vi "Alternating LEDs.vi"() -> ()   [LabVIEW 2014]
panel:
  in  "stop":bool
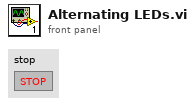
[diagram p1: front panel]
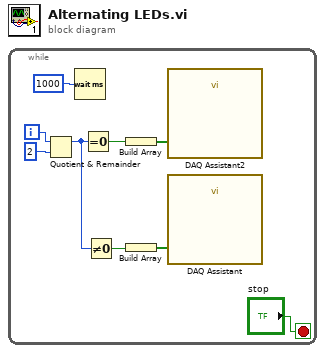
[diagram p0: block diagram]
diagram:
  n1 = while {
    i -> [w9]
    stop <- "stop" stop-if-true
    n2 = Quotient & Remainder(x=w9, y=2) -> (x-y*floor(x/y)=w3:i32)  [unwired: 1 out]
    n3 = Wait (ms)(milliseconds to wait=1000) -> ()  [unwired: 1 out]
    n4 = Equal To 0?(x=w3) -> (x = 0?=w2:bool)
    n5 = Not Equal To 0?(x=w3) -> (x != 0?=w1:bool)
    n6 = Build Array(w2) -> (w7:bool[])
    n7 = Build Array(w1) -> (w4:bool[])
    n8 = call "DAQ Assistant2"("data"=w7) -> ()  [unwired: 17 in, 2 out]
    n9 = call "DAQ Assistant"("data"=w4) -> ()  [unwired: 17 in, 2 out]
  }
